vi "音频分析（浮点）.vi"() -> ()   [LabVIEW 2015]
uses:
  <vilib>/sound2/lvsound2.llb/Sound Data Format.ctl
  <vilib>/sound2/lvsound2.llb/Sound File Write Open.vi
  <vilib>/sound2/lvsound2.llb/Sound File Write (SGL).vi
  <vilib>/measure/madcrms.llb/Basic Averaged DC-RMS for 1 Chan.vi
  <vilib>/measure/matone.llb/SINAD Analyzer 1 Chan.vi
  <vilib>/Analysis/NI_AALPro.lvlib
  <vilib>/measure/NI_MAPro.lvlib
panel:
  in  "文件类型":enum16{"wave", "裸数据"}(ring)
  in  "满量程幅度":sgl=2.8
  in  "输入衰减":sgl(ring)=1.0 items=["无衰减"=1, "五倍衰减"=5]
  out "文件长度":i32
  in  "分析长度":i32=10000
  in  "初始偏移":i32=10000
  in  "采样率":u32(ring)=48000 items=["192k"=192000, "96k"=96000, "48k"=48000]
  in  "分析通道":u16(ring) items=["左声道", "右声道"]
  in  "原始文件路径":path
  out "RMS value":dbl caption="均方根电压(V)" format="%0.2p"
  out "SINAD (dB)":dbl format="%.2p"
  out "detected fundamental\nfrequency":dbl caption="检测出的基频" format="%.2p"
  in  "wav文件路径 2":path caption="裸数据文件生成路径"
  in  "放大系数":sgl=1.0 format="%#_6f"
  in  "使能数据转换":bool
  in  "wav文件路径":path caption="wav文件生成路径"
  out "分析通道频谱(dBV)":T1(graph)
  out "左声道":sgl[](graph)
  out "分析通道导数":dbl[](graph)
  out "右声道":sgl[](graph)
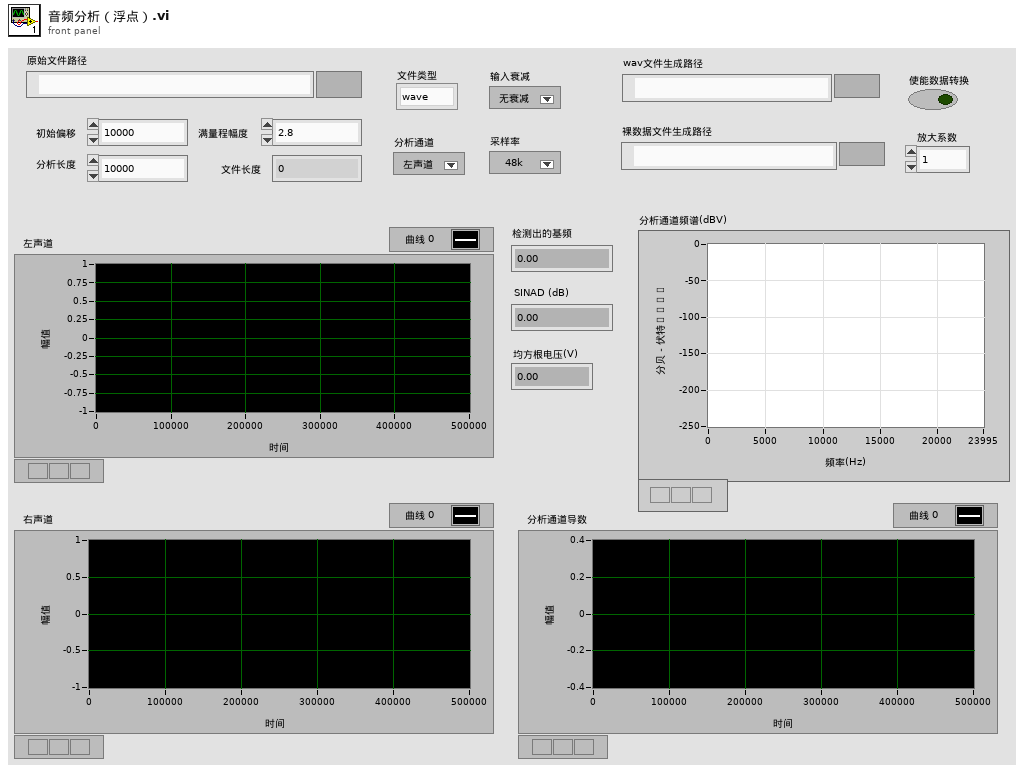
[diagram p1: front panel]
types:
  T1 = cluster{"f0":dbl, "df":dbl, "dB Spectrum (Hann)":dbl[]}
  T2 = enum16{"big-endian, network order", "native, host order", "little-endian"}
  T3 = enum16{"open", "replace", "create", "open or create", "replace or create", "replace or create with confirmation"}
  T4 = enum16{"Rectangular (none)", "Hanning", "Low side lobe"}
  T5 = enum16{"none", "input signal", "fundamental signal", "residual signal"}
  T6 = typedef "Sound Data Format.ctl" = cluster{"sample rate (S/s)":dbl, "number of channels":i32, "bits per sample":i32}
  T7 = typedef "Sound File Refnum.ctl" = refnum<file>
  T8 = cluster{"exported time signal":waveform(dbl), "exported spectrum (dB)":cluster{"f0":dbl, "df":dbl, "dB Spectrum (Hann)":dbl[]}}
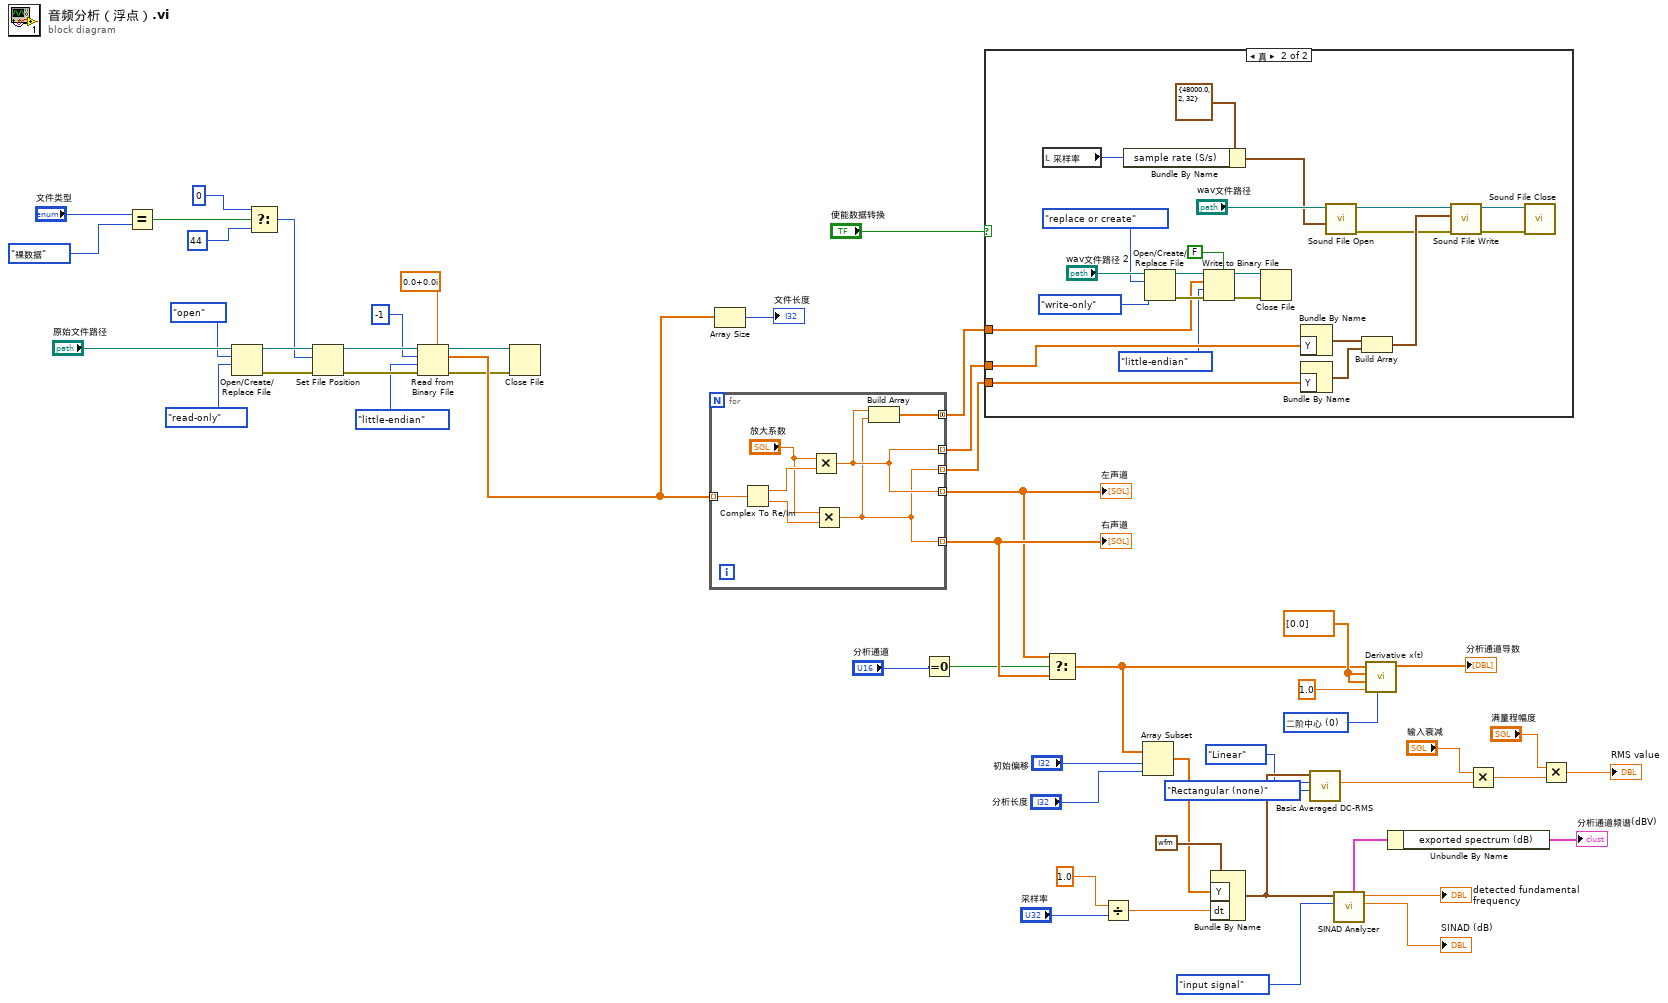
[diagram p0: block diagram]
diagram:
  w49 = u16 0 items=["二阶中心", "四阶中心", "前向", "后向"] ("method")
  w52 = dbl[] [0.0] ("Initial Condition")
  n1 = Equal?(x="文件类型", y=enum16{"wave", "裸数据"}."裸数据" ("文件类型")) -> (x = y?=w4:bool)
  n2 = Open/Create/Replace File(file path (use dialog)="原始文件路径", operation (0:open)=T3."open" ("操作(0:open)"), access (0:read/write)=enum16{"read/write", "read-only", "write-only"}."read-only" ("权限(0:read/write)")) -> (refnum out=w13:refnum<file>, error out=w12:errorcluster)  [unwired: 3 in, 1 out]
  n3 = Select(t=i64 0 ("偏移量（字节）（0）"), s=w4, f=i64 44 ("偏移量（字节）（0）")) -> (s? t:f=w1:i64)
  n4 = Set File Position(offset (in bytes) (0)=w1, refnum=w13, error in=w12) -> (refnum out=w11:refnum<file>, error out=w10:errorcluster)  [unwired: 1 in]
  n5 = Read from Binary File(5:csg 0.0+0.0i, 8:w10, 9:T2."little-endian" ("字节顺序(0:big-endian, network order)"), 10:-1 ("总数(1)"), 11:w11) -> (0:w5:errorcluster, 2:w18:csg[], 3:w6:refnum<file>)  [unwired: 1 in, 1 out]
  n6 = Close File(refnum=w6, error in=w5) -> ()  [unwired: 2 out]
  n7 = for {
    tunnel: w18 -> [w60] mode=indexing
    tunnel: [w56] -> w31 mode=indexing
    tunnel: [w55] -> w41 mode=indexing
    tunnel: [w56] -> w30 mode=indexing
    tunnel: [w55] -> w29 mode=indexing
    tunnel: [w54] -> w27 mode=concatenating
    n8 = Complex To Re/Im(x + iy=w60) -> (x=w59:sgl, y=w58:sgl)
    n9 = Multiply(x="放大系数", y=w59) -> (x*y=w56:sgl)
    n10 = Multiply(x="放大系数", y=w58) -> (x*y=w55:sgl)
    n11 = Build Array(w56, w55) -> (w54:sgl[])
  }
  "右声道" <- w41
  "左声道" <- w31
  n12 = Array Size(array=w18) -> (size(s)=→"文件长度":i32)
  n13 = Equal To 0?(x="分析通道") -> (x = 0?=w38:bool)
  n14 = case shown="真" "使能数据转换" {
    tunnel: w30 -> [_ w80]
    tunnel: w29 -> [_ w79]
    tunnel: w27 -> [_ w66]
    frame False {
    }
    frame True {
      n15 = local read "采样率"() -> (w76:u32)
      n16 = Bundle By Name(cluster=T6 {"sample rate (S/s)"=48000.0, "number of channels"=2, "bits per sample"=32} ("sound format"), "sample rate (S/s)"=w76) -> (w75:T6)
      n17 = Open/Create/Replace File(file path (use dialog)="wav文件路径 2", operation (0:open)=T3."replace or create" ("操作(0:open)"), access (0:read/write)=enum16{"read/write", "read-only", "write-only"}."write-only" ("权限(0:read/write)")) -> (refnum out=w63:refnum<file>, error out=w67:errorcluster)  [unwired: 3 in, 1 out]
      n18 = Write to Binary File(file (use dialog)=w63, data=w66, error in=w67, 5:FALSE ("预置数组或字符串大小？ (T)"), 9:T2."little-endian" ("字节顺序(0:big-endian, network order)")) -> (refnum out=w62:refnum<file>, error out=w61:errorcluster)  [unwired: 1 in, 1 out]
      n19 = Close File(refnum=w62, error in=w61) -> ()  [unwired: 2 out]
      n20 = Bundle By Name("Y"=w80) -> (w83:waveform(sgl))  [unwired: 1 in]
      n21 = Bundle By Name("Y"=w79) -> (w82:waveform(sgl))  [unwired: 1 in]
      n22 = call-poly <vilib>:"Sound File Open.vi"("sound format"=w75, "path"="wav文件路径") -> ("error out"=w73:errorcluster, "sound file refnum"=w74:T7)  [unwired: 8 in]
      n23 = Build Array(w83, w82) -> (w81:waveform(sgl)[])
      n24 = call-poly <vilib>:"Sound File Write.vi"("error in (no error)"=w73, "data"=w81, "sound file refnum"=w74) -> ("error out"=w71:errorcluster, "sound file refnum out"=w72:T7)  [unwired: 7 in]
      n25 = call <vilib>:"Sound File Close.vi"("error in (no error)"=w71, "sound file refnum"=w72) -> ()  [unwired: 9 in, 1 out]
    }
  }
  n26 = Select(t=w31, s=w38, f=w41) -> (s? t:f=w40:sgl[])
  n27 = Divide(x=1.0, y="采样率") -> (x/y=w35:dbl)
  n28 = Array Subset(array=w40, index="初始偏移", length="分析长度") -> (w42:sgl[])
  n29 = Bundle By Name(cluster=waveform(dbl) {"t0"=timestamp(0 s since 1904-01-01), "dt"=1.0, "Y"=[]} ("signal in"), "Y"=w42, "dt"=w35) -> (w26:waveform(dbl))
  n30 = call-poly <vilib>:"Basic Averaged DC-RMS.vi"("window"=T4."Rectangular (none)", "averaging type"=enum16{"Linear", "Exponential"}."Linear", "signal in"=w26) -> ("RMS value"=w22:dbl)  [unwired: 5 in, 3 out]
  n31 = call-poly <vilib>:"SINAD Analyzer.vi"("export  mode"=T5."input signal", "signal in"=w26) -> ("SINAD (dB)"=→"SINAD (dB)":dbl, "detected fundamental\nfrequency"=→"detected fundamental\nfrequency":dbl, "exported signals"=w44:T8)  [unwired: 4 in, 3 out]
  n32 = call <vilib>:"Derivative x(t).vi"("method"=w49, "dt"=1.0, "Final Condition"=w52, "Initial Condition"=w52, "X"=w40) -> ("dX/dt"=→"分析通道导数":dbl[])  [unwired: 5 in, 1 out]
  n33 = Unbundle By Name(w44) -> ("exported spectrum (dB)"=→"分析通道频谱(dBV)":T1)
  n34 = Multiply(x="输入衰减", y=w22) -> (x*y=w21:dbl)
  n35 = Multiply(x="满量程幅度", y=w21) -> (x*y=→"RMS value":dbl)
